vi "Read Configuration Filename.vi"(8 "error in (no error)":errorcluster, 11 "HGF_Configuration in":refnum<class "HGF_Configuration.lvclass">) -> (0 "error out":errorcluster, 2 "Configuration Filename":path, 3 "HGF_Configuration out":refnum<class "HGF_Configuration.lvclass">)   [LabVIEW 2012, in "HGF_ApplicationBaseClasses.lvlib" / "HGF_Configuration.lvclass"]
uses:
  HGF_Configuration.lvclass
  HGF_Configuration.lvclass/HGF_Configuration.ctl
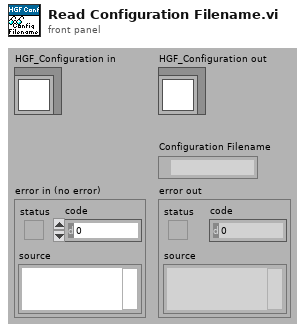
[diagram p1: front panel]
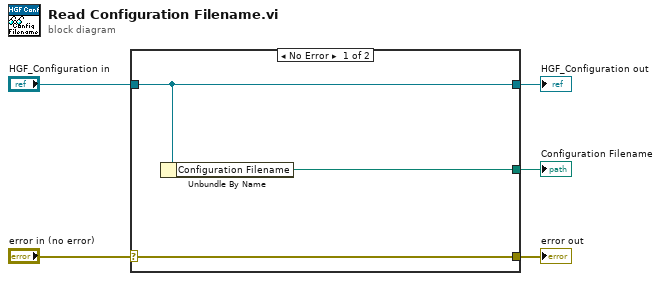
[diagram p0: block diagram]
diagram:
  n1 = case shown="No Error" "error in (no error)" {
    selector: "error in (no error)" -> [w8 w9]
    tunnel: [w8 w9] -> w4
    tunnel: [w7 w10] -> w2
    tunnel: "HGF_Configuration in" -> [w7 w10]
    tunnel: [w6 _] -> w1
    frame No Error {
      n2 = Unbundle By Name(w7) -> ("Configuration Filename"=w6:path)
    }
    frame Error {
    }
  }
  "error out" <- w4
  "HGF_Configuration out" <- w2
  "Configuration Filename" <- w1
